vi "Low_Pass_Filter.vi"(5 "Cut-Off Frequency":dbl, 6 "Sampling Interval":dbl, 8 "Previous Output":dbl, 10 "Previous Input":dbl, 11 "Current Input":dbl) -> (3 "Derivative":dbl)   [LabVIEW 2022 SP3]
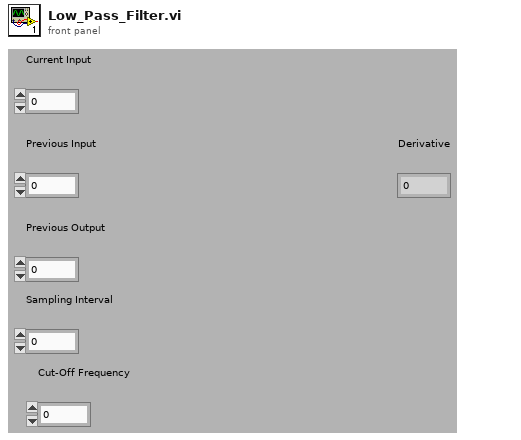
[diagram p1: front panel]
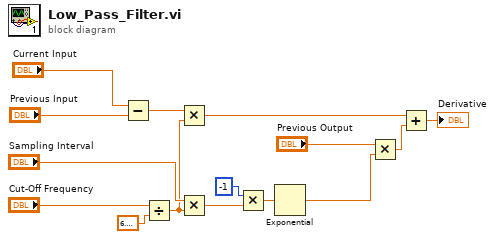
[diagram p0: block diagram]
diagram:
  n1 = Subtract(x="Current Input", y="Previous Input") -> (x-y=w2:dbl)
  n2 = Divide(x="Cut-Off Frequency", y=6.283185307179586) -> (x/y=w1:dbl)
  n3 = Multiply(x=w2, y=w1) -> (x*y=w3:dbl)
  n4 = Multiply(x="Sampling Interval", y=w1) -> (x*y=w12:dbl)
  n5 = Multiply(x=-1, y=w12) -> (x*y=w10:dbl)
  n6 = Exponential(1:w10) -> (0:w6:dbl)
  n7 = Multiply(x="Previous Output", y=w6) -> (x*y=w5:dbl)
  n8 = Add(x=w3, y=w5) -> (x+y=→"Derivative":dbl)
